vi "Device Test.vi"() -> ()   [LabVIEW 2011, in "Mass Flow Controller.lvclass"]
uses:
  Mass Flow Controller.lvclass
  Valve Status.ctl
  Aalborg GFC17/Aalborg GFC17.lvclass
panel:
  out "Flow Rate":dbl=0.17952059999999997
  in  "Valve Status":T1
  out "error out":errorcluster
  in  "Flow Rate Setpoing":dbl=50.0
  in  "stop":bool
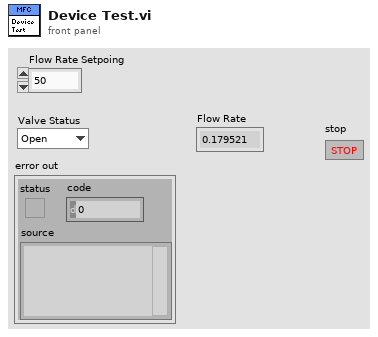
[diagram p1: front panel]
types:
  T1 = typedef "Mass Flow Controller.lvclass/Valve Status.ctl" = enum16{"Open", "Closed"}
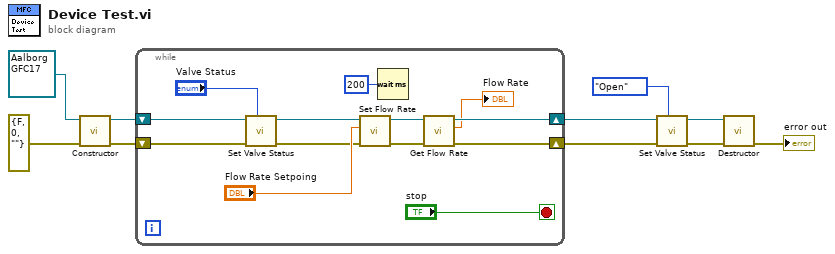
[diagram p0: block diagram]
diagram:
  n1 = call-dynamic "Constructor.vi"("error in (no error)"=errorcluster {"status"=FALSE, "code"=0, "source"=""}, "Aalborg GFC17 in"=refnum<class "Aalborg GFC17.lvclass"> refnum ("Aalborg GFC17.lvclass")) -> ("error out"=w1:errorcluster, "Aalborg GFC17 out"=w2:refnum<class "Aalborg GFC17.lvclass">)  [unwired: 7 in, 1 out]
  n2 = while {
    shift-right: [w12] -> w6
    shift-left: w1 -> [w19]
    shift-right: [w13] -> w7
    shift-left: w2 -> [w17]
    stop <- "stop" stop-if-true
    n3 = call-dynamic "Set Valve Status.vi"("Valve Status"="Valve Status", "error in (no error)"=w19, "Aalborg GFC17 in"=w17) -> ("error out"=w18:errorcluster, "Aalborg GFC17 out"=w16:refnum<class "Aalborg GFC17.lvclass">)  [unwired: 7 in]
    n4 = call-dynamic "Set Flow Rate.vi"("error in (no error)"=w18, "Flow Rate"="Flow Rate Setpoing", "Aalborg GFC17 in"=w16) -> ("error out"=w15:errorcluster, "Aalborg GFC17 out"=w14:refnum<class "Aalborg GFC17.lvclass">)  [unwired: 7 in]
    n5 = Wait (ms)(milliseconds to wait=u32 200) -> ()  [unwired: 1 out]
    n6 = call-dynamic "Get Flow Rate.vi"("error in (no error)"=w15, "Aalborg GFC17 in"=w14) -> ("error out"=w12:errorcluster, "Flow Rate"=→"Flow Rate":dbl, "Aalborg GFC17 out"=w13:refnum<class "Aalborg GFC17.lvclass">)  [unwired: 6 in, 1 out]
  }
  n7 = call-dynamic "Set Valve Status.vi"("Valve Status"=Valve_Status."Open", "error in (no error)"=w6, "Aalborg GFC17 in"=w7) -> ("error out"=w5:errorcluster, "Aalborg GFC17 out"=w4:refnum<class "Aalborg GFC17.lvclass">)  [unwired: 7 in]
  n8 = call-dynamic "Destructor.vi"("error in (no error)"=w5, "Aalborg GFC17 in"=w4) -> ("error out"=→"error out":errorcluster)  [unwired: 8 in, 1 out]
